vi "SERIAL_Open.vi"(7 "Serial Port (MXP)":T1=enum."MXP TTL", 10 "Update Rate (4Hz-60Hz)":u8=50, 11 "Nav6Mode (YPR)":T2) -> (0 "error out":errorcluster, 1 "Opened":bool, 3 "navX Ref":T3={"SerialPortRef"={"DevStatus"={"status"=FALSE, "code"=0, "source"=""}, "Serial Port Name"=""}, "Board Information"={"WhoAmI (50 | 0x32)"=0, "Board Revision"=0, "Firmware Major Version"=0, "Firmware Minor Version"=0, "NAVX_BOARD_CAPABILITY"={"OMNIMOUNT"=FALSE, "YAW_RESET"=FALSE, "VEL_AND_DISP"=FALSE}, "NAVX_BOARD_YAW_AXIS"={"BOARD_YAW_AXIS_UP"=FALSE, "BOARD_YAW_AXIS"=0}}, "Status"={"Update Rate Hz"=0, "Accelerometer Full-Scale Range"=0, "Gyro Full-Scale Range"=0, "NAVX_OP_STATUS"=0, "NAVX_CAL_STATUS"=0, "NAVX_SELFTEST_STATUS"=0, "NAVX_SENSOR_STATUS"={"MOVING"=FALSE, "YAW_STABLE"=FALSE, "MAG_DISTURBANCE"=FALSE, "ALTITUDE_VALID"=FALSE, "SEALEVEL_PRESS_SET"=FALSE, "FUSED_HEADING_VALID"=FALSE}}, "Offsets"={"Yaw"=0.0, "Quat W"=0.0, "Quat X"=0.0, "Quat Y"=0.0, "Quat Z"=0.0}, "Update Rate (4Hz-60Hz)"=50, "Nav6Mode (YPR)"=enum."YPR", "refnum name"="", "error"={"status"=FALSE, "code"=0, "source"=""}, "Loop VI Refnum"=refnum} {"Status"."NAVX_OP_STATUS" items=["INITIALIZING", "SELFTEST_IN_PROGRESS", "ERROR", "IMU_AUTOCAL_IN_PROGRESS", "NORMAL"]; "Status"."NAVX_CAL_STATUS" items=["IMU_CAL_STATE_MASK"=3, "IMU_CAL_INPROGRESS"=0, "IMU_CAL_ACCUMULATE"=1, "IMU_CAL_COMPLETE"=2, "MAG_CAL_COMPLETE"=4, "BARO_CAL_COMPLETE"=8]})   [LabVIEW 2015, in "navX-MXP IMU.lvlib"]
uses:
  navX-MXP IMU.lvlib
  Internal/navX Serial DevRef.ctl
  <vilib>/Rock Robotics/WPI/SerialPort/WPI_SerialPortRef.ctl
  COMMON/TypeDefs/Data TypeDefs/navX Board Information.ctl
  COMMON/TypeDefs/Value TypeDefs/navX NAVX_BOARD_CAPABILITY.ctl
  COMMON/TypeDefs/Value TypeDefs/navX NAVX_BOARD_YAW_AXIS.ctl
  COMMON/TypeDefs/Data TypeDefs/navX Status Data.ctl
  COMMON/TypeDefs/Value TypeDefs/navX NAVX_OP_STATUS.ctl
  COMMON/TypeDefs/Value TypeDefs/navX NAVX_CAL_STATUS.ctl
  COMMON/TypeDefs/Value TypeDefs/navX NAVX_SENSOR_STATUS.ctl
  TypeDefs/navX Serial Mode.ctl
  NI WPI/WPI_SerialPort_USB.ctl
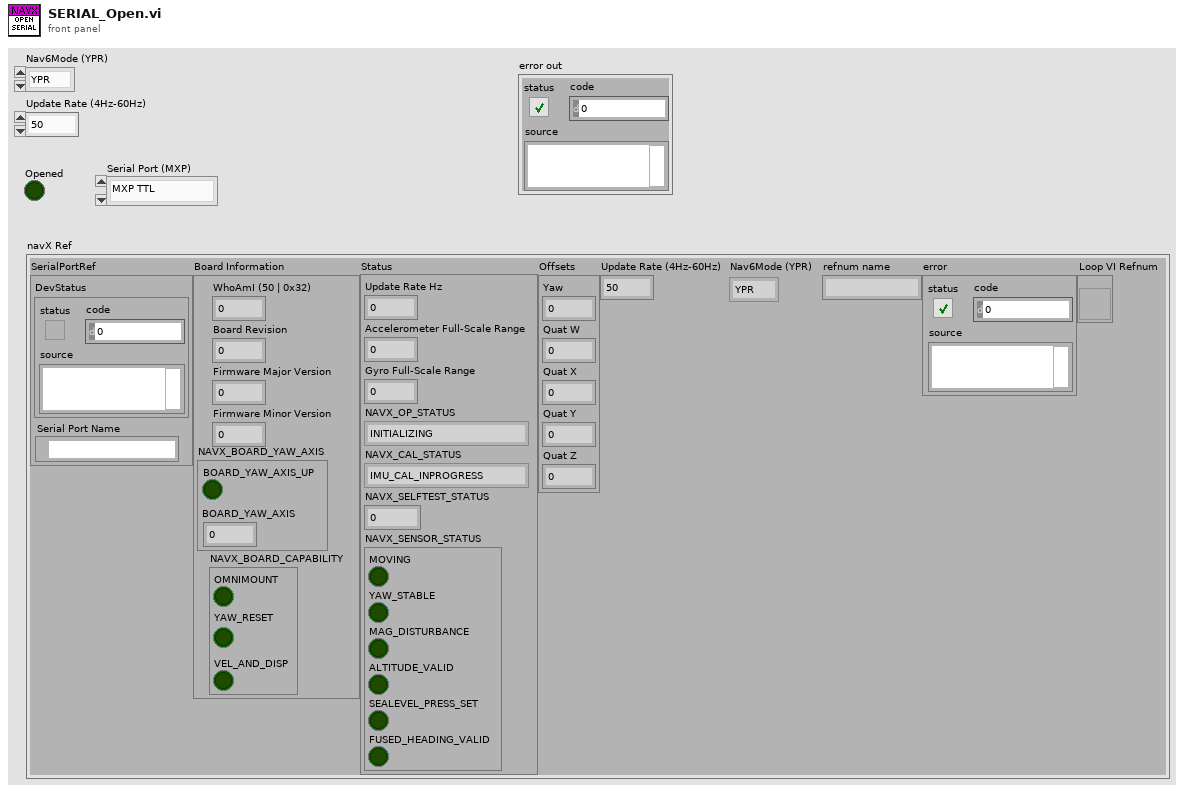
[diagram p1: front panel]
types:
  T1 = typedef "navX-MXP IMU.lvlib/WPI_SerialPort_USB.ctl" = enum16{"Onboard RS-232", "MXP TTL", "USB"}
  T2 = typedef "navX-MXP IMU.lvlib/navX Serial Mode.ctl" = enum16{"YPR", "Gyro", "Quaternion"}
  T3 = typedef "navX-MXP IMU.lvlib/navX Serial DevRef.ctl" = cluster{"SerialPortRef":T4, "Board Information":T5, "Status":T8, "Offsets":cluster{"Yaw":dbl, "Quat W":dbl, "Quat X":dbl, "Quat Y":dbl, "Quat Z":dbl}, "Update Rate (4Hz-60Hz)":u8, "Nav6Mode (YPR)":T2, "refnum name":string, "error":errorcluster, "Loop VI Refnum":refnum<vi>}
  T4 = typedef "WPI_SerialPortRef.ctl" = cluster{"DevStatus":errorcluster, "Serial Port Name":refnum<visa-resource-name>}
  T5 = typedef "navX-MXP IMU.lvlib/navX Board Information.ctl" = cluster{"WhoAmI (50 | 0x32)":u8, "Board Revision":u8, "Firmware Major Version":u8, "Firmware Minor Version":u8, "NAVX_BOARD_CAPABILITY":T6, "NAVX_BOARD_YAW_AXIS":T7}
  T6 = typedef "navX-MXP IMU.lvlib/navX NAVX_BOARD_CAPABILITY.ctl" = cluster{"OMNIMOUNT":bool, "YAW_RESET":bool, "VEL_AND_DISP":bool}
  T7 = typedef "navX-MXP IMU.lvlib/navX NAVX_BOARD_YAW_AXIS.ctl" = cluster{"BOARD_YAW_AXIS_UP":bool, "BOARD_YAW_AXIS":u8}
  T8 = typedef "navX-MXP IMU.lvlib/navX Status Data.ctl" = cluster{"Update Rate Hz":u8, "Accelerometer Full-Scale Range":u8, "Gyro Full-Scale Range":u16, "NAVX_OP_STATUS":T9, "NAVX_CAL_STATUS":T10, "NAVX_SELFTEST_STATUS":u8, "NAVX_SENSOR_STATUS":T11}
  T9 = typedef "navX-MXP IMU.lvlib/navX NAVX_OP_STATUS.ctl" = u8
  T10 = typedef "navX-MXP IMU.lvlib/navX NAVX_CAL_STATUS.ctl" = u8
  T11 = typedef "navX-MXP IMU.lvlib/navX NAVX_SENSOR_STATUS.ctl" = cluster{"MOVING":bool, "YAW_STABLE":bool, "MAG_DISTURBANCE":bool, "ALTITUDE_VALID":bool, "SEALEVEL_PRESS_SET":bool, "FUSED_HEADING_VALID":bool}
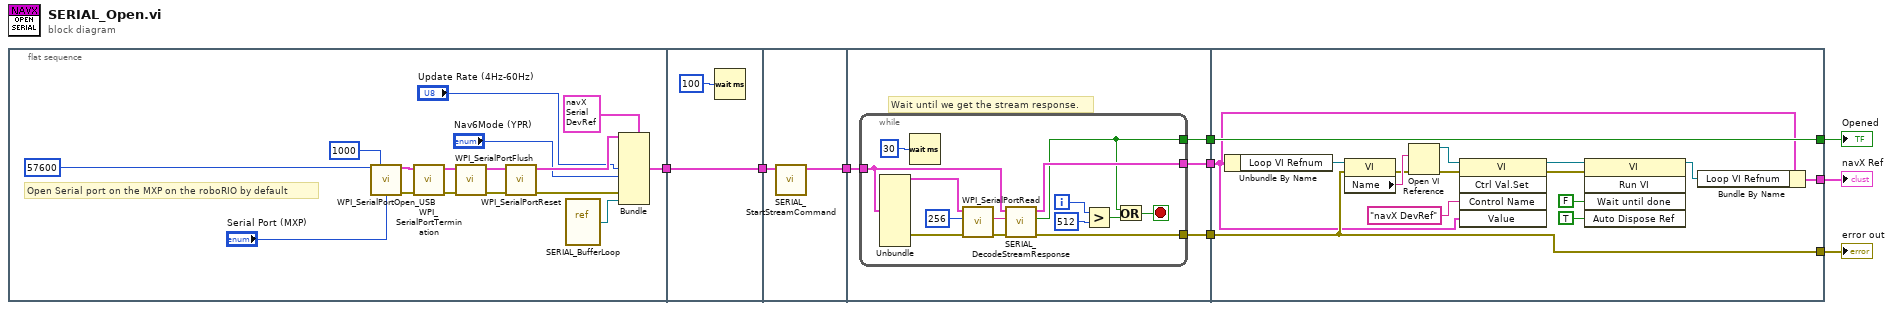
[diagram p0: block diagram]
diagram:
  n1 = flat-sequence {
    tunnel: [w19] -> w9
    tunnel: w9 -> [w27]
    tunnel: [w27] -> w8
    tunnel: w8 -> [w29]
    tunnel: [w28] -> w7
    tunnel: w7 -> [w31]
    tunnel: [w33] -> w3
    tunnel: [w32] -> w2
    tunnel: [w30] -> w1
    tunnel: [w62] -> w5
    tunnel: [w58] -> w6
    tunnel: [w54] -> w4
    tunnel: w3 -> [w51]
    tunnel: w2 -> [w58]
    tunnel: w1 -> [w62]
    frame #0 {
      # "Open Serial port on the MXP on the roboRIO by default"
      n2 = call "WPI_SerialPortOpen_USB.vi"("Baud Rate"=u32 57600, "Timeout Value (ms)"=u32 1000, "Serial Port"="Serial Port (MXP)") -> ("SerialPortRef"=w11:T4, "error out"=w10:errorcluster)  [unwired: 11 in]
      n3 = call <vilib>:"WPI_SerialPortTermination.vi"("error in (no error)"=w10, "SerialPortRef"=w11) -> ("error out"=w25:errorcluster, "SerialPortRef"=w24:T4)  [unwired: 8 in]
      n4 = call <vilib>:"WPI_SerialPortFlush.vi"("error in (no error)"=w25, "SerialPortRef"=w24) -> ("error out"=w23:errorcluster, "SerialPortRef"=w22:T4)  [unwired: 8 in]
      n5 = call <vilib>:"WPI_SerialPortReset.vi"("error in (no error)"=w23, "SerialPortRef"=w22) -> ("error out"=w16:errorcluster, "SerialPortRef"=w20:T4)  [unwired: 8 in]
      n6 = vi-ref "SERIAL_BufferLoop.vi"() -> (w15:refnum<vi>)
      n7 = Bundle(cluster=T3 {"SerialPortRef"={"DevStatus"={"status"=FALSE, "code"=0, "source"=""}, "Serial Port Name"=""}, "Board Information"={"WhoAmI (50 | 0x32)"=0, "Board Revision"=0, "Firmware Major Version"=0, "Firmware Minor Version"=0, "NAVX_BOARD_CAPABILITY"={"OMNIMOUNT"=FALSE, "YAW_RESET"=FALSE, "VEL_AND_DISP"=FALSE}, "NAVX_BOARD_YAW_AXIS"={"BOARD_YAW_AXIS_UP"=FALSE, "BOARD_YAW_AXIS"=0}}, "Status"={"Update Rate Hz"=0, "Accelerometer Full-Scale Range"=0, "Gyro Full-Scale Range"=0, "NAVX_OP_STATUS"=0, "NAVX_CAL_STATUS"=0, "NAVX_SELFTEST_STATUS"=0, "NAVX_SENSOR_STATUS"={"MOVING"=FALSE, "YAW_STABLE"=FALSE, "MAG_DISTURBANCE"=FALSE, "ALTITUDE_VALID"=FALSE, "SEALEVEL_PRESS_SET"=FALSE, "FUSED_HEADING_VALID"=FALSE}}, "Offsets"={"Yaw"=0.0, "Quat W"=0.0, "Quat X"=0.0, "Quat Y"=0.0, "Quat Z"=0.0}, "Update Rate (4Hz-60Hz)"=50, "Nav6Mode (YPR)"=enum."YPR", "refnum name"="", "error"={"status"=FALSE, "code"=0, "source"=""}, "Loop VI Refnum"=refnum} ("navX Ref Object"), "SerialPortRef"=w20, "Update Rate (4Hz-60Hz)"="Update Rate (4Hz-60Hz)", "Nav6Mode (YPR)"="Nav6Mode (YPR)", "error"=w16, "Loop VI Refnum"=w15) -> (w19:T3)  [unwired: 4 in]
    }
    frame #1 {
      n8 = Wait (ms)(milliseconds to wait=u32 100) -> ()  [unwired: 1 out]
    }
    frame #2 {
      n9 = call "SERIAL_StartStreamCommand.vi"("navX Ref"=w29) -> ("navX Ref"=w28:T3)  [unwired: 10 in]
    }
    frame #3 {
      # "Wait until we get the stream response."
      n10 = while {
        tunnel: [w44] -> w33
        tunnel: [w43] -> w32
        tunnel: w31 -> [w41]
        tunnel: [w39] -> w30
        i -> [w38]
        stop <- w36 stop-if-true
        n11 = Unbundle(w41) -> ("SerialPortRef"=w47:T4, "error"=w42:errorcluster)  [unwired: 7 out]
        n12 = Wait (ms)(milliseconds to wait=u32 30) -> ()  [unwired: 1 out]
        n13 = call <vilib>:"WPI_SerialPortRead.vi"("error in (no error)"=w42, "Num Bytes to Read"=u32 256, "SerialPortRef"=w47) -> ("error out"=w45:errorcluster, "Buffer"=w40:string)  [unwired: 6 in, 1 out]
        n14 = call "SERIAL_DecodeStreamResponse.vi"("error in"=w45, "Buffer"=w40, "navX DevRef"=w41) -> ("error out"=w43:errorcluster, "Valid"=w39:bool, "navX DevRef"=w44:T3)  [unwired: 6 in]
        n15 = Greater?(x=w38, y=512) -> (0:w35:bool)
        n16 = Or(x=w39, y=w35) -> (x .or. y?=w36:bool)
      }
    }
    frame #4 {
      n17 = Unbundle By Name(w51) -> ("Loop VI Refnum"=w61:refnum<vi>)
      n18 = property class="VI"(reference=w61, error in=w58) -> (error out=w59:errorcluster, "Name"=w60:string)  [unwired: 1 out]
      n19 = Open VI Reference(vi path=w60, error in (no error)=w59) -> (vi reference=w53:refnum<vi>, error out=w49:errorcluster)  [unwired: 4 in]
      n20 = invoke class="VI" method="Ctrl Val.Set"(reference=w53, error in=w49, "Control Name"="navX DevRef", "Value"=w51) -> (reference out=w50:refnum<vi>, error out=w48:errorcluster)  [unwired: 1 in, 3 out]
      n21 = invoke class="VI" method="Run VI"(reference=w50, error in=w48, "Wait until done"=FALSE ("Wait Until Done"), "Auto Dispose Ref"=TRUE ("Auto Dispose Reference")) -> (reference out=w55:refnum<vi>)  [unwired: 1 in, 4 out]
      n22 = Bundle By Name(cluster=w51, "Loop VI Refnum"=w55) -> (w54:T3)
    }
  }
  "error out" <- w6
  "navX Ref" <- w4
  "Opened" <- w5
